vi "ConvertToGray_IfNecessary.vi"(10 "Image Type":T1 items=["Grayscale (U8)", "Grayscale (I16)", "Grayscale (SGL)", "Complex (CSG)", "RGB (U32)", "HSL (U32)", "RGB (U64)", "Grayscale (U16)"], 11 "Image in":u32[][](array[numeric])) -> (3 "Image out":u32[][](array[numeric]))   [LabVIEW 2017, in "ImageAcquisitionLibrary.lvlib"]
uses:
  ImageAcquisitionLibrary.lvlib
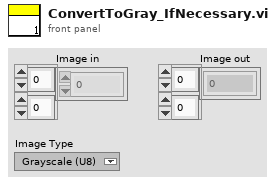
[diagram p1: front panel]
types:
  T1 = typedef "Image Type" = u32
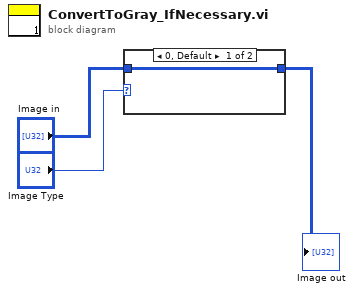
[diagram p0: block diagram]
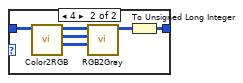
[diagram p2: hidden frame]
diagram:
  n1 = case shown="0, Default" "Image Type" {
    tunnel: "Image in" -> [w4 w10]
    tunnel: [w4 w5] -> w2
    frame 0, Default {
    }
    frame 4 {
      n2 = call "Color2RGB.vi"("Image Pixels (U32)"=w10) -> ("Array 3"=w7:u8[][], "Array"=w8:u8[][], "Array 2"=w9:u8[][])  [unwired: 8 in]
      n3 = call "RGB2Gray.vi"("Blue"=w7, "Green"=w8, "Red"=w9) -> ("Array out"=w6:u8[][])  [unwired: 8 in]
      n4 = To Unsigned Long Integer(number=w6) -> (unsigned 32bit integer=w5:u32[][])
    }
  }
  "Image out" <- w2
